vi "IMMU - Read Accelerometer & Gyro.vi"(6 "dt":dbl=0.01 format="%0.2f", 7 "Reset Gyro":bool, 8 "error in (no error)":errorcluster, 9 "Gyro Offset Array In":i16[](array[numeric]), 10 "Accel Offset Array In":i16[](array[numeric]), 11 "I2C Ref In":T1={"myRIO Reference"={"myRIO Model"=enum."Unknown", "myRIO Hardware Reference"={"Generic FPGA Reference"=refnum, "Allow multiple opens"=FALSE}}, "I2C Channels Enum"=enum."Not Connected", "I2C Configuration"={"I2C Transfer Rate"=enum."Fast mode (400 kbps)"}}) -> (0 "error out":errorcluster, 1 "Gyro Rotation Out (degrees)":dbl[](array[numeric]), 2 "Gyro Rotational Velocity Out (deg/s)":dbl[](array[numeric]), 3 "Output Acceleration Array (ms^2)":dbl[](array[numeric]), 5 "I2C Ref Out":T1={"myRIO Reference"={"myRIO Model"=enum."Unknown", "myRIO Hardware Reference"={"Generic FPGA Reference"=refnum, "Allow multiple opens"=FALSE}}, "I2C Channels Enum"=enum."Not Connected", "I2C Configuration"={"I2C Transfer Rate"=enum."Fast mode (400 kbps)"}})   [LabVIEW 2021]
uses:
  <vilib>/myRIO/Instrument Drivers/Onboard IO/I2C/typedefs/I2C Reference.ctl
  <vilib>/myRIO/Common/Instrument Driver Framework/Utilities/typedefs/myRIO Generic Hardware Reference.ctl
  <vilib>/myRIO/Common/Instrument Driver Framework/Utilities/typedefs/Hardware Version Enum.ctl
  <vilib>/myRIO/Common/Instrument Driver Framework/Utilities/typedefs/myRIO v1.0 Reference.ctl
  <vilib>/myRIO/Common/Instrument Driver Framework/Utilities/typedefs/Generic FPGA Reference.ctl
  <vilib>/myRIO/Common/Instrument Driver Framework/myRIO v1.0/I2C/typedefs/I2C Channels Enum.ctl
  <vilib>/myRIO/Instrument Drivers/Onboard IO/I2C/typedefs/I2C Configuration.ctl
  <vilib>/myRIO/Instrument Drivers/Onboard IO/I2C/typedefs/I2C Transfer Rate.ctl
  <vilib>/Utility/error.llb/Error Cluster From Error Code.vi
  <vilib>/myRIO/Common/Instrument Driver Framework/myRIO v1.0/I2C/vis/myRIO v1.0 Write I2C.vi
  <vilib>/myRIO/Common/Instrument Driver Framework/myRIO v1.0/I2C/vis/myRIO v1.0 Read I2C.vi
  <vilib>/myRIO/Instrument Drivers/Onboard IO/I2C/I2C.lvlib
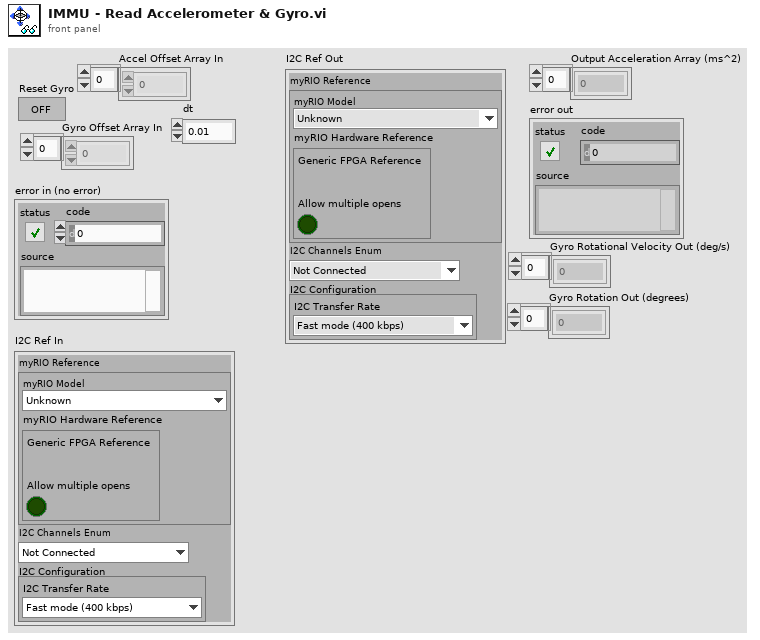
[diagram p1: front panel]
types:
  T1 = typedef "I2C.lvlib/I2C Reference.ctl" = cluster{"myRIO Reference":T2, "I2C Channels Enum":T6, "I2C Configuration":T7}
  T2 = typedef "myRIO Generic Hardware Reference.ctl" = cluster{"myRIO Model":T3, "myRIO Hardware Reference":T4}
  T3 = typedef "Hardware Version Enum.ctl" = enum16{"Unknown", "myRIO-1900", "myRIO-1950", "roboRIO", "NI ELVIS RIO CM", "ELVIS III"}
  T4 = typedef "myRIO v1.0 Reference.ctl" = cluster{"Generic FPGA Reference":T5, "Allow multiple opens":bool}
  T5 = typedef "Generic FPGA Reference.ctl" = refnum<k20>
  T6 = typedef "I2C Channels Enum.ctl" = enum16{"Not Connected", "A/I2C", "B/I2C", "I2C/I2C"}
  T7 = typedef "I2C.lvlib/I2C Configuration.ctl" = cluster{"I2C Transfer Rate":T8}
  T8 = typedef "I2C.lvlib/I2C Transfer Rate.ctl" = enum16{"Standard mode (100 kbps)", "Fast mode (400 kbps)"}
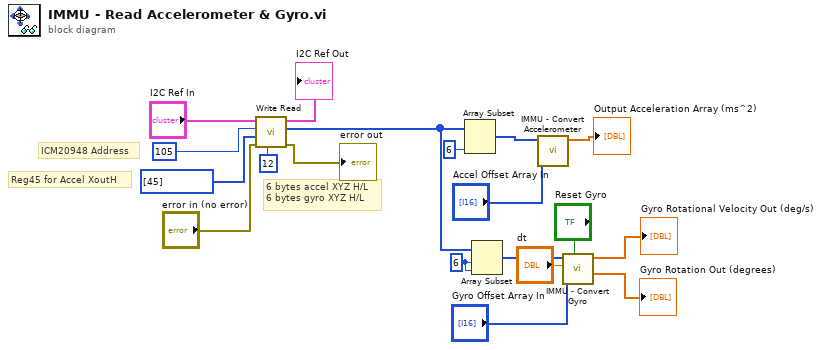
[diagram p0: block diagram]
diagram:
  w17 = 6 ("index")
  # "6 bytes accel XYZ H/L\n6 bytes gyro XYZ H/L"
  # "Reg45 for Accel XoutH"
  # "ICM20948 Address"
  n1 = call <vilib>:"Write Read.vi"("Byte Count"=u32 12, "error in (no error)"="error in (no error)", "Bytes to Write"=u8[] [45], "Slave Address (7-bit)"=u8 105, "I2C Ref In"="I2C Ref In") -> ("error out"=→"error out":errorcluster, "Bytes Read"=w10:u8[], "I2C Ref Out"=→"I2C Ref Out":T1)  [unwired: 3 in]
  n2 = Array Subset(array=w10, length=6) -> (w9:u8[])  [unwired: 1 in]
  n3 = Array Subset(array=w10, index=w17, length=w17) -> (w16:u8[])
  n4 = call "IMMU - Convert Accelerometer.vi"("Accel Offset Array In"="Accel Offset Array In", "Input Raw Accel Array (U8)"=w9) -> ("Output Acceleration Array (ms^2)"=→"Output Acceleration Array (ms^2)":dbl[])  [unwired: 9 in]
  n5 = call "IMMU - Convert Gyro.vi"("initialize"="Reset Gyro", "Offset Array In"="Gyro Offset Array In", "dt"="dt", "Gyro Data Array In"=w16) -> ("Gyro Rotation Out (degrees)"=→"Gyro Rotation Out (degrees)":dbl[], "Gyro Rotational Velocity Out (deg/s)"=→"Gyro Rotational Velocity Out (deg/s)":dbl[])  [unwired: 6 in]
